vi "Actor Core.vi"(8 "error in":errorcluster, 11 "IMAQdx Cam Actor in":refnum<class "IMAQdx Cam Actor.lvclass">) -> (0 "error out":errorcluster, 3 "Actor out":refnum<class "Actor.lvclass">)   [LabVIEW 2014, in "IMAQdx Cam Actor.lvlib" / "IMAQdx Cam Actor.lvclass"]
doc: "(<B>Filename</B>: Actor Framework.lvlib:Actor.lvclass:Actor Core.vi)\n\nReceives messages to the actor, reacts to them, and initiates any error handling that may shut the actor down.\n\nDescendant classes may override this VI to append parallel tasks for the actor to complete while it handles messages. Overrides use the Call Parent Method node."
uses:
  IMAQdx Cam Actor.lvclass
  <vilib>/ActorFramework/Actor/Actor.lvclass
  <vilib>/userdefined/High Color/IMAQdx.ctl
  <vilib>/vision/Image Controls.llb/IMAQ Image.ctl
  IMAQdx Cam Actor.lvclass/IMAQdx Cam Actor.ctl
  <vilib>/ActorFramework/Actor/Actor.lvclass/Actor.ctl
  <vilib>/ActorFramework/Message Enqueuer/Message Enqueuer.lvclass/Message Enqueuer.ctl
  IMAQdx Cam Actor Messages/New Image Msg/New Image Msg.lvclass/New Image Msg.ctl
  <vilib>/ActorFramework/Message Enqueuer/Init from Existing Queue.vi
  <vilib>/ActorFramework/Message Enqueuer/Enqueue.vi
  <vilib>/ActorFramework/Message Priority Queue/Priority Enqueue.vi
  <vilib>/ActorFramework/Message Enqueuer/Message Enqueuer.lvclass
  IMAQdx Cam Actor Messages/New Image Msg/New Image Msg.lvclass
panel:
  in  "Image":T1
  in  "Frame Done":refnum<event-registration>
  in  "Stop":bool
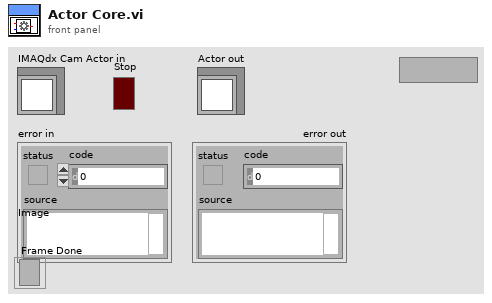
[diagram p1: front panel]
types:
  T1 = typedef "IMAQ Image.ctl" = refnum<image>
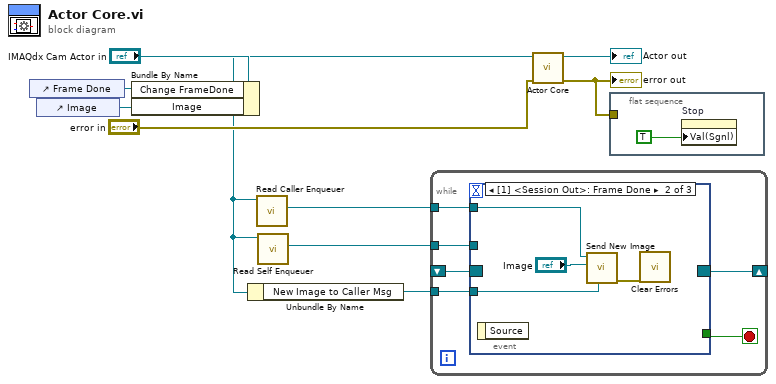
[diagram p0: block diagram]
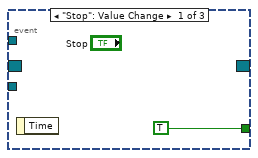
[diagram p2: hidden frame]
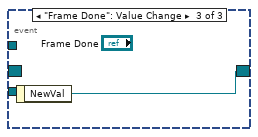
[diagram p3: hidden frame]
diagram:
  n1 = control-ref of="Frame Done"() -> (w2:refnum<vi>)
  n2 = control-ref of="Image"() -> (w1:refnum<vi>)
  n3 = Bundle By Name(cluster="IMAQdx Cam Actor in", "Change FrameDone"=w2, "Image"=w1) -> (w4:refnum<class "IMAQdx Cam Actor.lvclass">)
  n4 = Unbundle By Name(w4) -> ("New Image to Caller Msg"=w5:refnum<class "New Image Msg.lvclass">)
  n5 = call <vilib>:"Read Caller Enqueuer.vi"("Actor"=w4) -> ("Caller Enqueuer"=w3:refnum<class "Message Enqueuer.lvclass">)  [unwired: 10 in]
  n6 = call <vilib>:"Read Self Enqueuer.vi"("Actor"=w4) -> ("Self Enqueuer"=w7:refnum<class "Message Enqueuer.lvclass">)  [unwired: 10 in]
  n7 = while {
    tunnel: w7 -> [w15]
    shift-right: [w13] -> _
    shift-left: _ -> [w14]
    tunnel: w5 -> [w12]
    tunnel: w3 -> [w11]
    stop <- w16 stop-if-true
    n8 = event shown="[1] <Session Out>: Frame Done" {
      selector: w14 -> [_ _ _]
      dyn-events: [_ _ w22] -> w13
      timeout: _ -> [_ _ _]
      tunnel: [TRUE _ _] -> w16
      tunnel: w15 -> [_ _ _]
      tunnel: w12 -> [_ w19 _]
      tunnel: w11 -> [_ w21 _]
      event "Stop": Value Change {
        n9 = event-data() -> ()  [unwired: 1 in, 1 out]
      }
      event event #0x0 {
        n10 = event-data() -> ()  [unwired: 1 in, 1 out]
        n11 = call "Send New Image.vi"("Msg Type"=w19, "Image"="Image", "Message Enqueuer"=w21) -> ("error out"=w20:errorcluster)  [unwired: 7 in, 1 out]
        n12 = call <vilib>:"Clear Errors.vi"("error in (no error)"=w20) -> ()  [unwired: 5 in, 2 out]
      }
      event "Frame Done": Value Change {
        n13 = event-data() -> ("NewVal"=w22:refnum<event-registration>)  [unwired: 1 in]
      }
    }
  }
  n14 = call-parent "Actor Core.vi"("error in"="error in", "Actor in"=w4) -> ("error out"=w8:errorcluster, "Actor out"=→"Actor out":refnum<class "Actor.lvclass">)  [unwired: 8 in]
  "error out" <- w8
  n15 = flat-sequence {
    tunnel: w8 -> [_]
    frame #0 {
      n16 = property on="Stop" class="Bool (strict)"("Val(Sgnl)"=TRUE) -> ()  [unwired: 2 in, 2 out]
    }
  }
